vi "tcp_get_trace_data.vi"(0 "connection_id_in":refnum<k5>, 1 "button_tcp_get_trace":bool, 5 "sva_ready_in":bool, 9 "tcp_connected_in":bool, 11 "error in":errorcluster) -> (4 "connection_id_out":refnum<k5>, 6 "sva_ready_out":bool, 10 "tcp_connected_out":bool, 13 "trace_data":string, 14 "new_data_available":bool, 15 "error out":errorcluster)   [LabVIEW 2025]
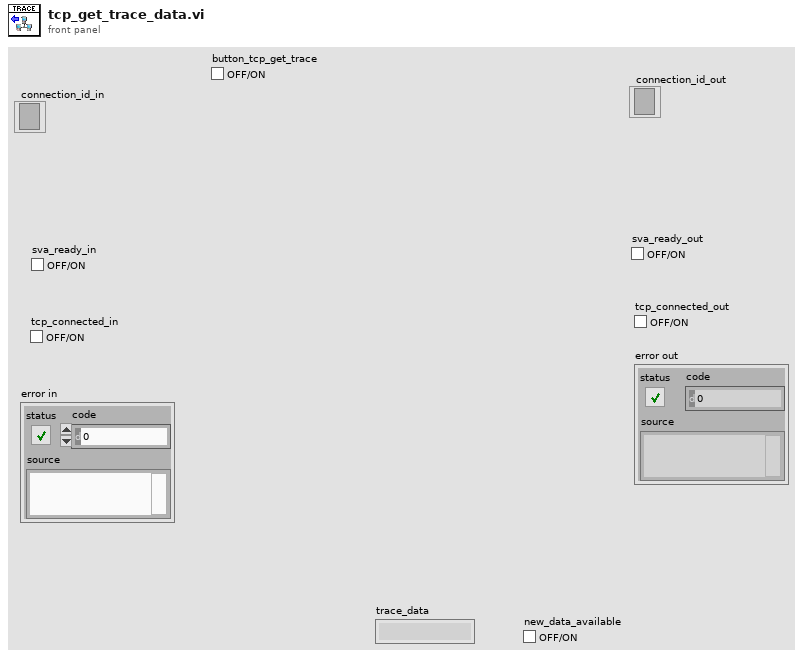
[diagram p1: front panel]
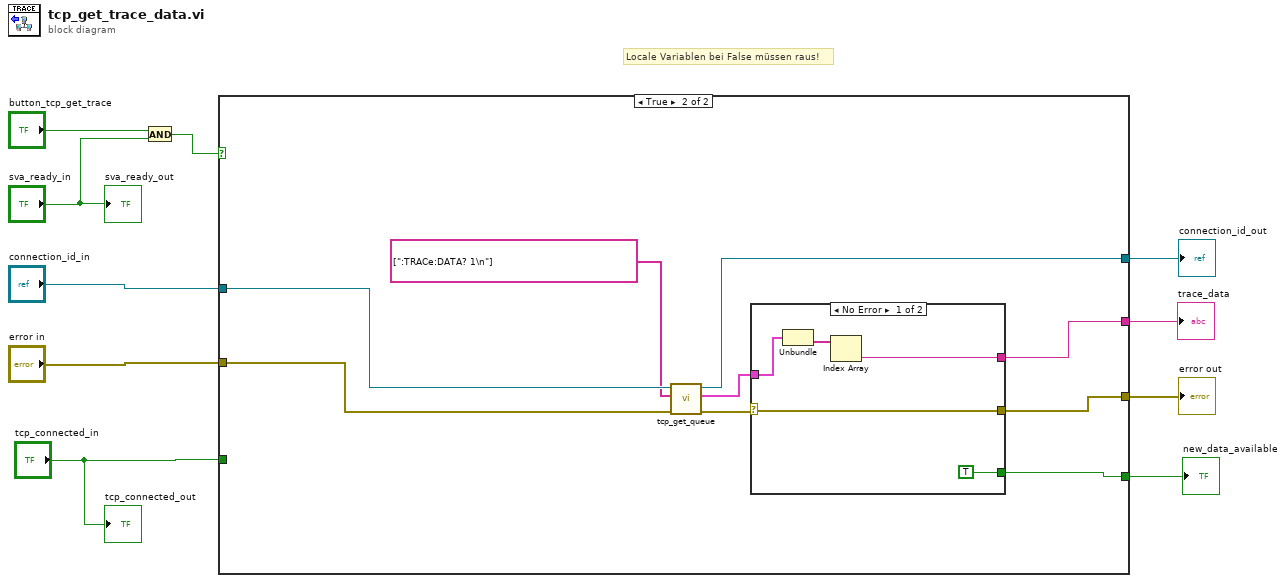
[diagram p0: block diagram]
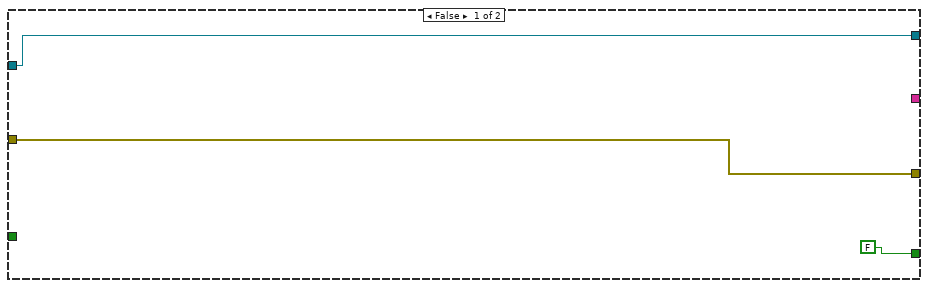
[diagram p2: hidden frame]
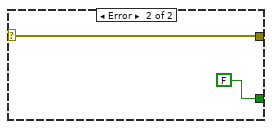
[diagram p3: hidden frame]
diagram:
  # "Locale Variablen bei False müssen raus!"
  n1 = And(x="button_tcp_get_trace", y="sva_ready_in") -> (x .and. y?=w10:bool)
  n2 = case shown="True" w10 {
    tunnel: [w11 w18] -> w8
    tunnel: [w13 w19] -> w7
    tunnel: "connection_id_in" -> [w13 w17]
    tunnel: "error in" -> [w11 w16]
    tunnel: "tcp_connected_in" -> [_ _]
    tunnel: [FALSE ("tcp_connected_in") w20] -> w4
    tunnel: [_ w14] -> w1
    frame False {
    }
    frame True {
      n3 = call "tcp_get_queue.vi"("error in"=w16, "command queue"=string[] [":TRACe:DATA? 1\n"], "connection in"=w17) -> ("error out"=w22:errorcluster, "output"=w21:cluster{string[], string[]}, "connection out"=w19:refnum<k5>)  [unwired: 6 in]
      n4 = case shown="No Error" w22 {
        selector: w22 -> [w24 w28]
        tunnel: w21 -> [w27 _]
        tunnel: [TRUE FALSE] -> w20
        tunnel: [w24 w28] -> w18
        tunnel: [w23 _] -> w14
        frame No Error {
          n5 = Unbundle(w27) -> (w26:string[])  [unwired: 1 out]
          n6 = Index Array(array=w26) -> (element=w23:string)  [unwired: 1 in]
        }
        frame Error {
        }
      }
    }
  }
  "error out" <- w8
  "connection_id_out" <- w7
  "new_data_available" <- w4
  "trace_data" <- w1
  "tcp_connected_out" <- "tcp_connected_in"
  "sva_ready_out" <- "sva_ready_in"
